vi "Set Interval.vi"(8 "error in (no error)":errorcluster, 10 "Interval (ms)":dbl, 11 "Synchronization Device in":refnum<class "Sync Device.lvclass">) -> (0 "error out":errorcluster, 3 "Synchronization Device out":refnum<class "Sync Device.lvclass">)   [LabVIEW 2023, in "Sync Device.lvlib" / "Sync Device.lvclass"]
uses:
  Sync Device.lvclass
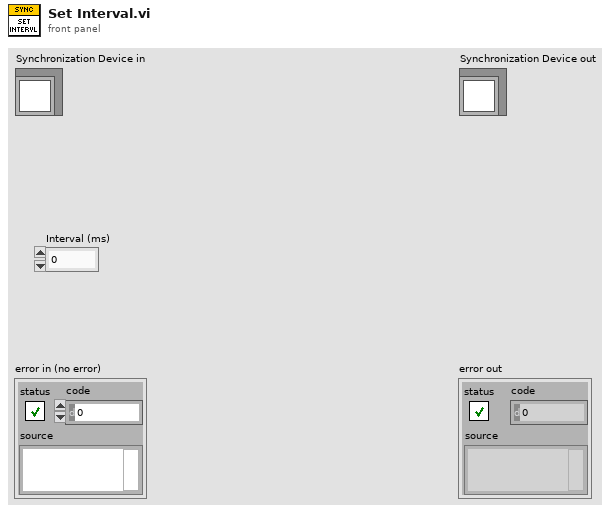
[diagram p1: front panel]
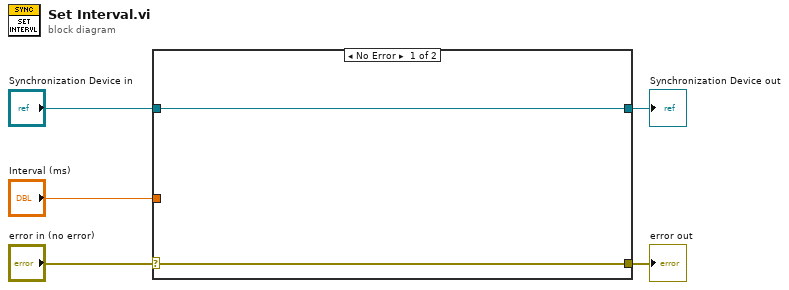
[diagram p0: block diagram]
diagram:
  n1 = case shown="No Error" "error in (no error)" {
    selector: "error in (no error)" -> [w6 w9]
    tunnel: [w6 w9] -> w4
    tunnel: [w7 w8] -> w2
    tunnel: "Synchronization Device in" -> [w7 w8]
    tunnel: "Interval (ms)" -> [_ _]
    frame No Error {
    }
    frame Error {
    }
  }
  "error out" <- w4
  "Synchronization Device out" <- w2
